vi "TestHelper_FilePacketInfo.vi"(11 "Number of Bytes":i32=4) -> (0 "Packet Data":u8[](array[numeric]), 1 "File ID":string, 2 "Packet Number":i32, 3 "Last Packet?":bool)   [LabVIEW 2017]
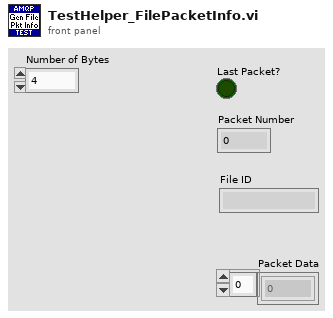
[diagram p1: front panel]
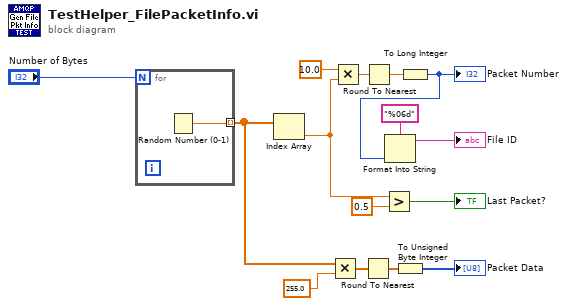
[diagram p0: block diagram]
diagram:
  n1 = for {
    N: "Number of Bytes" -> [_]
    tunnel: [w16] -> w7 mode=indexing
    n2 = Random Number (0-1)() -> (number: 0 to 1=w16:dbl)
  }
  n3 = Index Array(array=w7) -> (element=w9:dbl)  [unwired: 1 in]
  n4 = Multiply(x=w7, y=255.0 ("x")) -> (x*y=w5:dbl[])
  n5 = Multiply(x=10.0, y=w9) -> (x*y=w2:dbl)
  n6 = Round To Nearest(number=w5) -> (nearest integer value=w4:dbl[])
  n7 = Round To Nearest(number=w2) -> (nearest integer value=w14:dbl)
  n8 = Greater?(x=w9, y=0.5) -> (0:→"Last Packet?":bool)
  n9 = To Unsigned Byte Integer(number=w4) -> (unsigned 8bit integer=→"Packet Data":u8[])
  n10 = To Long Integer(number=w14) -> (32bit integer=w1:i32)
  "Packet Number" <- w1
  n11 = Format Into String(format string="%06d", w1) -> (resulting string=→"File ID":string)  [unwired: 2 in, 1 out]
